vi "addRemDisList.vi"(11 "Pixel Status":T1) -> (3 "Disabled Pixels":u8[](array[numeric]))   [LabVIEW 2018]
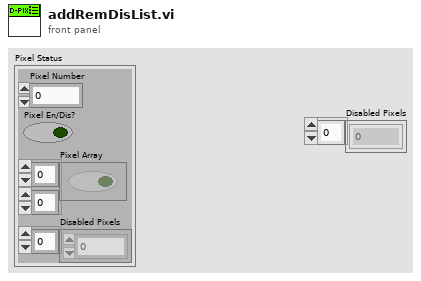
[diagram p1: front panel]
types:
  T1 = cluster{"Pixel Number":u16, "Pixel En/Dis?":bool, "Pixel Array":bool[][], "Disabled Pixels":u8[]}
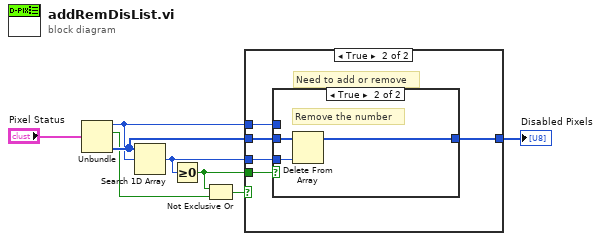
[diagram p0: block diagram]
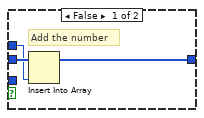
[diagram p3: hidden frame]
diagram:
  n1 = Unbundle("Pixel Status") -> ("Pixel Number"=w2:u16, "Pixel En/Dis?"=w3:bool, "Disabled Pixels"=w4:u8[])  [unwired: 1 out]
  n2 = Search 1D Array(1D array=w4, element=w2) -> (index of element=w7:i32)  [unwired: 1 in]
  n3 = Greater Or Equal To 0?(x=w7) -> (x >= 0?=w6:bool)
  n4 = Not Exclusive Or(1:w3, 2:w6) -> (0:w5:bool)
  n5 = case shown="True" w5 {
    tunnel: w6 -> [_ w14]
    tunnel: w4 -> [w9 w13]
    tunnel: w7 -> [_ w12]
    tunnel: w2 -> [_ w11]
    tunnel: [w9 w10] -> w1
    frame False {
      # "Do Nothing to the list"
    }
    frame True {
      # "Need to add or remove"
      n6 = case shown="True" w14 {
        tunnel: w13 -> [w17 w20]
        tunnel: w12 -> [_ w19]
        tunnel: w11 -> [w16 _]
        tunnel: [w15 w18] -> w10
        frame False {
          # "Add the number"
          n7 = Insert Into Array(array=w17, new element=w16) -> (w15:u8[])  [unwired: 1 in]
        }
        frame True {
          # "Remove the number"
          n8 = Delete From Array(array=w20, index=w19) -> (array with subset deleted=w18:u8[])  [unwired: 1 in, 1 out]
        }
      }
    }
  }
  "Disabled Pixels" <- w1
